vi "Struct Get.vi"(5 "use temporary file? (F)":bool, 6 "reinit cluster to default (false)":bool, 7 "cluster ref (empty)":refnum<vi>, 8 "error in":errorcluster, 10 "variable":string, 11 "GOLPI ref in":T3={"pipe handle"={"lv_proc.dll file path"=path "", "process instance handle"=[], "debug mode"=FALSE, "debug data"=[]}, "fast read timeout [ms]"=500, "fast read settle time [ms]"=10, "fast read to multiple [ms]"=1, "max elements per input line"=100, "slow read timeout [ms]"=5000, "stdin double format specifier"="%_16e", "max elements per stdout output column"=100, "console mode bitstream"=FALSE, "bitstream first read timeout [ms]"=1000, "bitstream read timeout [ms]"=50, "struct transfer possible"=FALSE}) -> (0 "error out":errorcluster, 2 "octave struct items":T1[](array[typedef]), 3 "GOLPI ref. out":T3={"pipe handle"={"lv_proc.dll file path"=path "", "process instance handle"=[], "debug mode"=FALSE, "debug data"=[]}, "fast read timeout [ms]"=500, "fast read settle time [ms]"=10, "fast read to multiple [ms]"=1, "max elements per input line"=100, "slow read timeout [ms]"=5000, "stdin double format specifier"="%_16e", "max elements per stdout output column"=100, "console mode bitstream"=FALSE, "bitstream first read timeout [ms]"=1000, "bitstream read timeout [ms]"=50, "struct transfer possible"=FALSE})   [LabVIEW 2013, in "GOLPI library.lvlib"]
doc: "This VI will use GOLPI package function 'golpi_conv_struct()' in GNU Octave to retrieve a structure in binary format. Then it will parse the binary data into the array of structure items. In next step it will try to assign the decoded items to the LV cluster if it is referenced. Optionally the LV cluster may be reinitialized to default before assigning its items. If reference to the cluster is not assigned this VI will just parse the binary octave data to array of structure items.\nThe whole function is made as recoursive so it should be able to assign struct withing struct and so on."
uses:
  GOLPI library.lvlib
  Public/GOLPI reference Type Def.ctl
  LV Process source distribution/Pipe Handle.ctl
  Type Definitions/Struct Item Record.ctl
  Type Definitions/Struct Item Types.ctl
  Type Definitions/Custom Error Codes Enum Type Def.vi
  Get Variable - polymorph parts/Get 1D Array Double.vi
  LV Process source distribution/LV Process library.lvlib
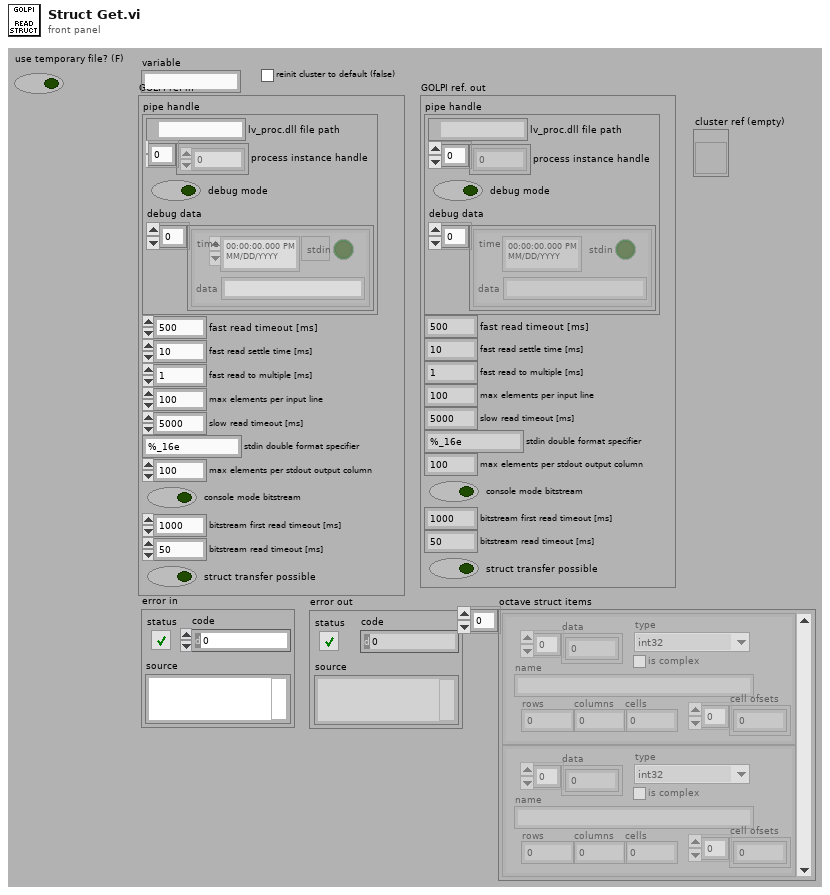
[diagram p1: front panel]
types:
  T1 = typedef "GOLPI library.lvlib/Struct Item Record.ctl" = cluster{"data":u8[], "type":T2, "name":string, "rows":i32, "columns":i32, "cells":i32, "is complex":bool, "cell ofsets":u32[]}
  T2 = typedef "GOLPI library.lvlib/Struct Item Types.ctl" = enum16{"int32", "uint32", "single", "double", "string", "cell array"}
  T3 = typedef "GOLPI library.lvlib/GOLPI reference Type Def.ctl" = cluster{"pipe handle":T4, "fast read timeout [ms]":u32, "fast read settle time [ms]":u32, "fast read to multiple [ms]":u32, "max elements per input line":u32, "slow read timeout [ms]":u32, "stdin double format specifier":string, "max elements per stdout output column":u32, "console mode bitstream":bool, "bitstream first read timeout [ms]":u32, "bitstream read timeout [ms]":u32, "struct transfer possible":bool}
  T4 = typedef "LV Process library.lvlib/Pipe Handle.ctl" = cluster{"lv_proc.dll file path":path, "process instance handle":u32[], "debug mode":bool, "debug data":cluster{"time":timestamp, "stdin":bool, "data":string}[]}
  T5 = typedef "GOLPI library.lvlib/Custom Error Codes Enum Type Def.vi" = enum16{"no error", "00 working directory PAR1 missing", "01 octave binary PAR1 missing", "02 octave report error PAR1", "03 empty output last cmd PAR1", "04 missing temporary file PAR1", "05 pwd PAR 1 not exist", "10 var PAR1 not string, vect", "11 var PAR1 not num, scal, ~compl", "12 var PAR1 not num, scal, compl", "13 var PAR1 not num, vect, ~compl", "14 var PAR1 not num, vect, compl", "15 var PAR1 not num, mat, ~compl", "16 var PAR1 not num, mat, ~compl", "30 read timeout", "60 bitstream transport failed", "61 bitstream decode error PAR1", "62 bitstream cannot be set", "70 struct transfer not possible", "99 not finished"}
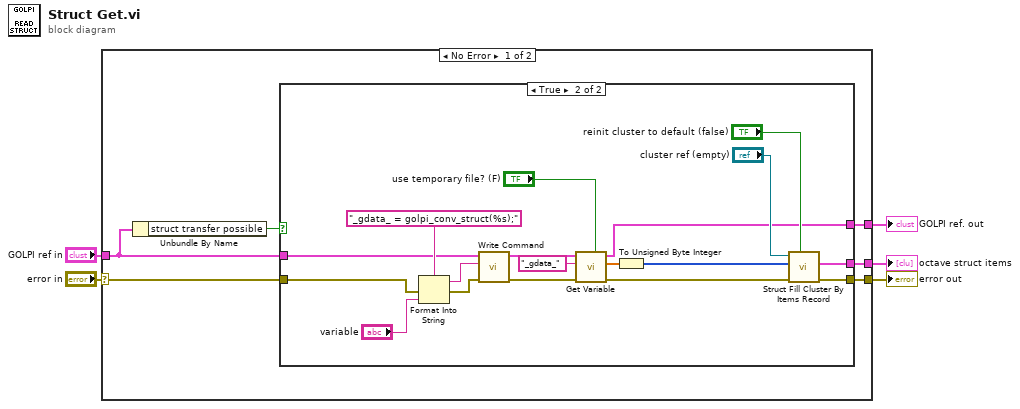
[diagram p0: block diagram]
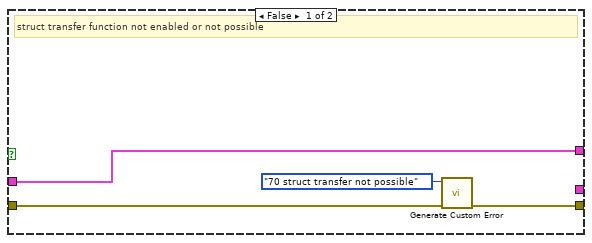
[diagram p2: hidden frame]
diagram:
  n1 = case shown="No Error" "error in" {
    selector: "error in" -> [w8 w35]
    tunnel: [w11 w35] -> w5
    tunnel: [w10 _] -> w4
    tunnel: "GOLPI ref in" -> [w9 w34]
    tunnel: [w7 w34] -> w1
    frame No Error {
      n2 = Unbundle By Name(w9) -> ("struct transfer possible"=w6:bool)
      n3 = case shown="True" w6 {
        tunnel: [w14 w27] -> w11
        tunnel: [_ w24] -> w10
        tunnel: w9 -> [w15 w18]
        tunnel: w8 -> [w13 w17]
        tunnel: [w15 w16] -> w7
        frame False {
          # "struct transfer function not enabled or not possible"
          n4 = call "Generate Custom Error.vi"("error in"=w13, "GOLPI error"=Custom_Error_Codes_Enum_Type_Def.vi."70 struct transfer not possible") -> ("error out"=w14:errorcluster)  [unwired: 9 in]
        }
        frame True {
          n5 = Format Into String(format string="_gdata_ = golpi_conv_struct(%s);", error in=w17, "variable") -> (resulting string=w33:string, error out=w21:errorcluster)  [unwired: 1 in]
          n6 = call "Write Command.vi"("error in"=w21, "command"=w33, "GOLPI ref. in"=w18) -> ("error out"=w19:errorcluster, "GOLPI ref. out"=w30:T3)  [unwired: 7 in]
          n7 = call-poly "Get Variable.vi"("use temporary file? (F)"="use temporary file? (F)", "error in"=w19, "variable name"="_gdata_", "GOLPI ref. in"=w30) -> ("error out"=w20:errorcluster, "value"=w28:dbl[], "GOLPI ref. out"=w16:T3)  [unwired: 5 in]
          n8 = To Unsigned Byte Integer(number=w28) -> (unsigned 8bit integer=w25:u8[])
          n9 = call "Struct Fill Cluster By Items Record.vi"("reinit cluster to default (false)"="reinit cluster to default (false)", "error in"=w20, "data in"=w25, "cluster ref (empty)"="cluster ref (empty)") -> ("error out"=w27:errorcluster, "octave struct out"=w24:T1[])  [unwired: 5 in, 1 out]
        }
      }
    }
    frame Error {
    }
  }
  "error out" <- w5
  "octave struct items" <- w4
  "GOLPI ref. out" <- w1
